vi "Generate Array Row 2016.vi"(6 "Cluster":T1, 9 "Feet of\nStainless to be\nUsed (Count)":i32, 10 "Flow":dbl, 11 "Zeroed Pressure":dbl format="%.2f") -> (2 "IK":dbl, 3 "Array":dbl[](array[numeric]))   [LabVIEW 2016]
uses:
  Waterloo DAQ/controls/Kpro hydraulic measurement cluster.ctl
  KPRO_lv2015/Kpro Globals.vi
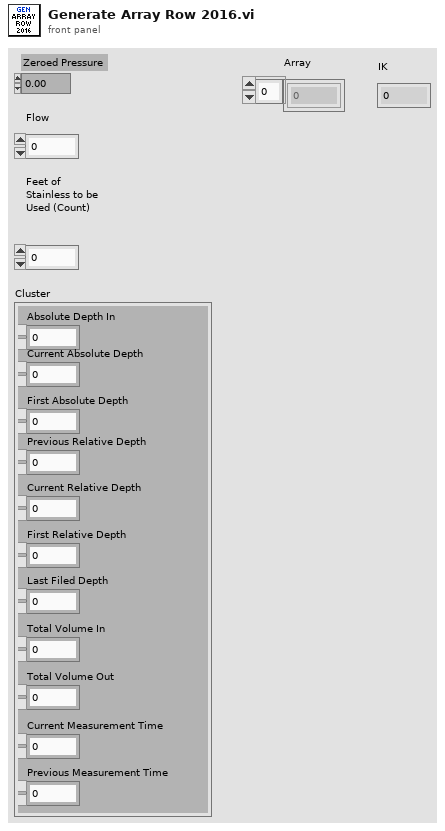
[diagram p1: front panel]
types:
  T1 = typedef "Kpro hydraulic measurement cluster.ctl" = cluster{"Absolute Depth In":dbl, "Current Absolute Depth":dbl, "First Absolute Depth":dbl, "Previous Relative Depth":dbl, "Current Relative Depth":dbl, "First Relative Depth":dbl, "Last Filed Depth":dbl, "Total Volume In":dbl, "Total Volume Out":dbl, "Current Measurement Time":dbl, "Previous Measurement Time":dbl}
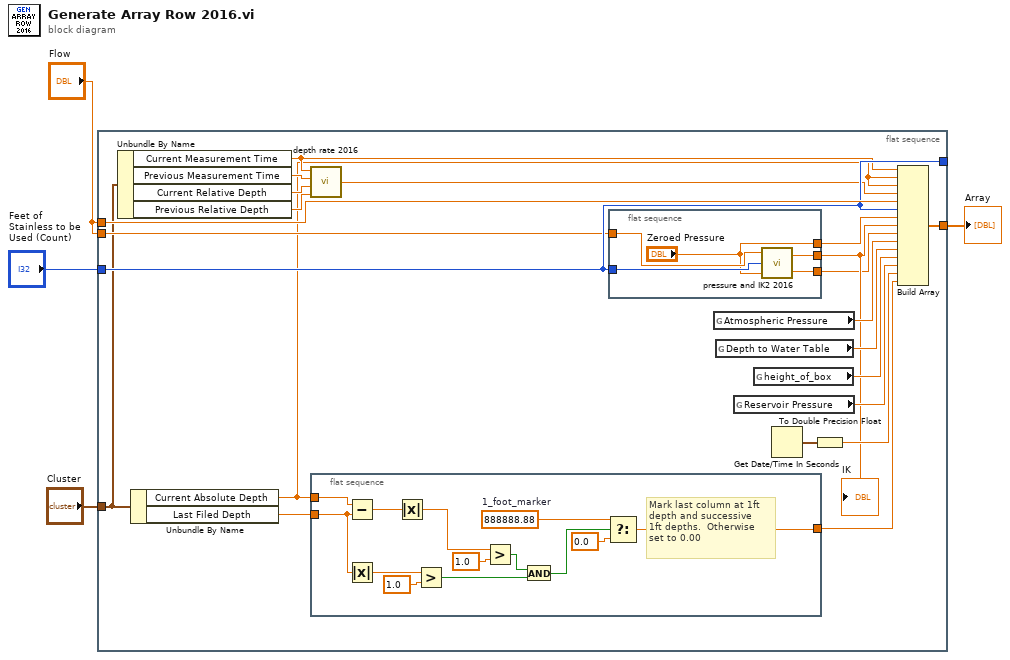
[diagram p0: block diagram]
diagram:
  n1 = flat-sequence {
    tunnel: [w26] -> w1
    tunnel: "Flow" -> [w25]
    tunnel: "Feet of\nStainless to be\nUsed (Count)" -> [w13]
    tunnel: "Cluster" -> [w8]
    tunnel: [w13] -> _
    tunnel: "Flow" -> [w12]
    frame #0 {
      n2 = Unbundle By Name(w8) -> ("Current Measurement Time"=w6:dbl, "Previous Measurement Time"=w9:dbl, "Current Relative Depth"=w10:dbl, "Previous Relative Depth"=w11:dbl)
      n3 = Unbundle By Name(w8) -> ("Current Absolute Depth"=w5:dbl, "Last Filed Depth"=w17:dbl)
      n4 = call "depth rate 2016.vi"("Depth Last"=w11, "Depth Current"=w10, "Time Last"=w9, "Time Current"=w6) -> ("Depth Rate"=w7:dbl)
      n5 = flat-sequence {
        tunnel: [w39] -> w19
        tunnel: w17 -> [w35]
        tunnel: w5 -> [w32]
        frame #0 {
          w41 = 888888.88  # 1_foot_marker
          # "Mark last column at 1ft \ndepth and successive\n1ft depths.  Otherwise\nset to 0.00"
          n6 = Subtract(x=w32, y=w35) -> (x-y=w44:dbl)
          n7 = Absolute Value(x=w35) -> (abs(x)=w33:dbl)
          n8 = Absolute Value(x=w44) -> (abs(x)=w42:dbl)
          n9 = Greater?(x=w33, y=1.0) -> (0:w36:bool)
          n10 = Greater?(x=w42, y=1.0) -> (0:w37:bool)
          n11 = And(x=w37, y=w36) -> (x .and. y?=w38:bool)
          n12 = Select(t=w41, s=w38, f=0.0) -> (s? t:f=w39:dbl)
        }
      }
      n13 = flat-sequence {
        tunnel: [w31] -> w14
        tunnel: ["Zeroed Pressure"] -> w16
        tunnel: w12 -> [w30]
        tunnel: [w29] -> w15
        tunnel: w13 -> [w28]
        frame #0 {
          n14 = call "pressure and IK2 2016.vi"("Pressure"="Zeroed Pressure", "Ft. of SS"=w28, "flow"=w30) -> ("Corrected Headloss"=w31:dbl, "IK"=w29:dbl)
        }
      }
      n15 = global read "Kpro Globals.vi" "Atmospheric Pressure"() -> (w24:dbl)
      n16 = global read "Kpro Globals.vi" "Depth to Water Table"() -> (w22:dbl)
      n17 = global read "Kpro Globals.vi" "Reservoir Pressure"() -> (w23:dbl)
      n18 = global read "Kpro Globals.vi" "height_of_box"() -> (w21:dbl)
      n19 = Get Date/Time In Seconds() -> (seconds since 1Jan1904=w18:timestamp)
      n20 = To Double Precision Float(number=w18) -> (double precision float=w20:dbl)
      n21 = Build Array(w6, w5, w5, w7, w25, w13, w16, w15, w14, w24, w22, w21, w23, w20, w19) -> (w26:dbl[])
      "IK" <- w15
    }
  }
  "Array" <- w1
